vi "Get Joystick 2016.vi"() -> (2 "Pilot-CoPilot Controls":T1)   [LabVIEW 2015]
uses:
  Subsystem VIs/Robot Control Outputs 2016.ctl
  Global Variables/refnum names.vi
  <vilib>/Rock Robotics/WPI/Utilities/WPI_GetSetVariantRefNum.vi
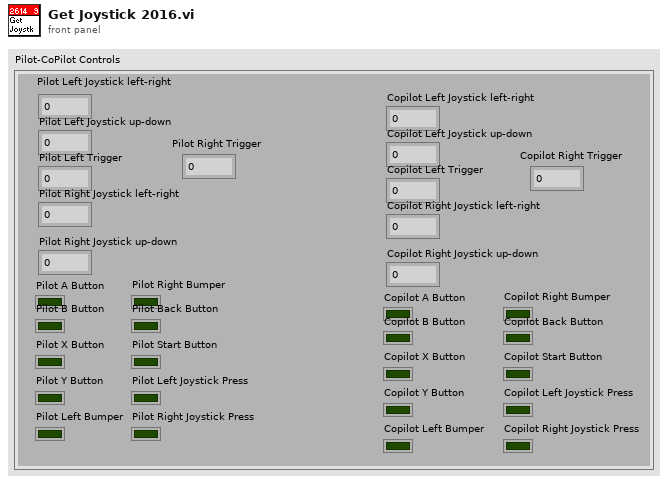
[diagram p1: front panel]
types:
  T1 = typedef "Robot Control Outputs 2016.ctl" = cluster{"Pilot Left Joystick left-right":dbl, "Pilot Left Joystick up-down":dbl, "Pilot A Button":bool, "Pilot B Button":bool, "Pilot X Button":bool, "Pilot Y Button":bool, "Pilot Left Bumper":bool, "Pilot Right Bumper":bool, "Pilot Back Button":bool, "Pilot Start Button":bool, "Pilot Left Joystick Press":bool, "Pilot Right Joystick Press":bool, "Pilot Left Trigger":dbl, "Pilot Right Joystick left-right":dbl, "Pilot Right Joystick up-down":dbl, "Pilot Right Trigger":dbl, "Copilot Left Joystick left-right":dbl, "Copilot Left Joystick up-down":dbl, "Copilot A Button":bool, "Copilot B Button":bool, "Copilot X Button":bool, "Copilot Y Button":bool, "Copilot Left Bumper":bool, "Copilot Right Bumper":bool, "Copilot Back Button":bool, "Copilot Start Button":bool, "Copilot Left Joystick Press":bool, "Copilot Right Joystick Press":bool, "Copilot Left Trigger":dbl, "Copilot Right Joystick left-right":dbl, "Copilot Right Joystick up-down":dbl, "Copilot Right Trigger":dbl}
  T2 = typedef "WPI_JoystickDevRef.ctl" = cluster{"Device":T3}
  T3 = typedef "WPI_JoystickDeviceEnum.ctl" = enum16{"USB 0", "USB 1", "USB 2", "USB 3", "USB 4", "USB 5"}
  T4 = cluster{"Axes[0]":dbl, "Axes[1]":dbl, "Axes[2]":dbl, "Axes[3]":dbl, "Axes[4]":dbl, "Axes[5]":dbl, "Axes[6]":dbl, "Axes[7]":dbl, "Axes[8]":dbl}
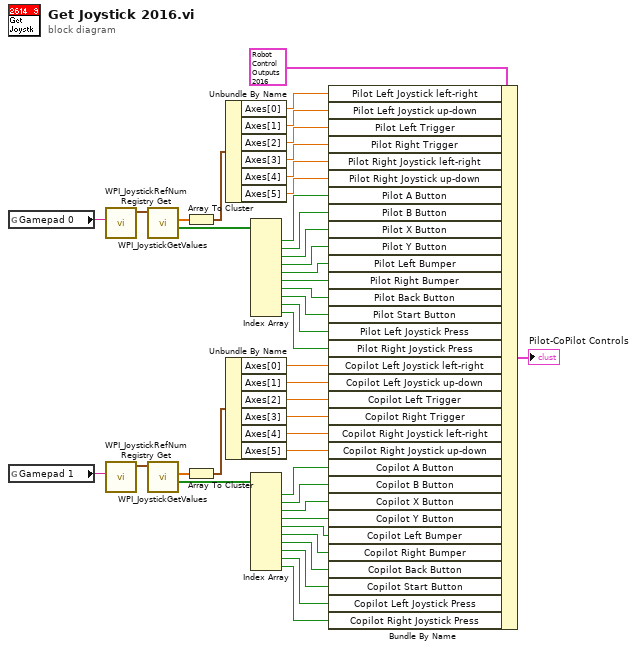
[diagram p0: block diagram]
diagram:
  n1 = global read "refnum names.vi" "Gamepad 0"() -> (w21:string)
  n2 = global read "refnum names.vi" "Gamepad 1"() -> (w20:string)
  n3 = call <vilib>:"WPI_JoystickRefNum Registry Get.vi"("refnum name"=w21) -> ("JoystickDevRef"=w42:T2)  [unwired: 9 in, 1 out]
  n4 = call <vilib>:"WPI_JoystickRefNum Registry Get.vi"("refnum name"=w20) -> ("JoystickDevRef"=w22:T2)  [unwired: 9 in, 1 out]
  n5 = call <vilib>:"WPI_JoystickGetValues.vi"("JoystickDevRef"=w42) -> ("Buttons"=w33:bool[], "Axes"=w41:dbl[])  [unwired: 6 in, 3 out]
  n6 = call <vilib>:"WPI_JoystickGetValues.vi"("JoystickDevRef"=w22) -> ("Buttons"=w18:bool[], "Axes"=w19:dbl[])  [unwired: 6 in, 3 out]
  n7 = Array To Cluster(array=w41) -> (cluster=w40:T4)
  n8 = Array To Cluster(array=w19) -> (cluster=w17:T4)
  n9 = Unbundle By Name(w40) -> ("Axes[0]"=w39:dbl, "Axes[1]"=w38:dbl, "Axes[2]"=w37:dbl, "Axes[3]"=w36:dbl, "Axes[4]"=w35:dbl, "Axes[5]"=w34:dbl)
  n10 = Unbundle By Name(w17) -> ("Axes[0]"=w16:dbl, "Axes[1]"=w15:dbl, "Axes[2]"=w14:dbl, "Axes[3]"=w13:dbl, "Axes[4]"=w12:dbl, "Axes[5]"=w11:dbl)
  n11 = Index Array(array=w33) -> (element #1=w32:bool, element #2=w31:bool, element #3=w30:bool, element #4=w29:bool, element #5=w28:bool, element #6=w27:bool, element #7=w26:bool, element #8=w25:bool, element #9=w24:bool, element #10=w23:bool)  [unwired: 10 in]
  n12 = Index Array(array=w18) -> (element #1=w10:bool, element #2=w9:bool, element #3=w8:bool, element #4=w7:bool, element #5=w5:bool, element #6=w6:bool, element #7=w4:bool, element #8=w3:bool, element #9=w2:bool, element #10=w1:bool)  [unwired: 10 in]
  n13 = Bundle By Name(cluster=T1 {"Pilot Left Joystick left-right"=0.0, "Pilot Left Joystick up-down"=0.0, "Pilot A Button"=FALSE, "Pilot B Button"=FALSE, "Pilot X Button"=FALSE, "Pilot Y Button"=FALSE, "Pilot Left Bumper"=FALSE, "Pilot Right Bumper"=FALSE, "Pilot Back Button"=FALSE, "Pilot Start Button"=FALSE, "Pilot Left Joystick Press"=FALSE, "Pilot Right Joystick Press"=FALSE, "Pilot Left Trigger"=0.0, "Pilot Right Joystick left-right"=0.0, "Pilot Right Joystick up-down"=0.0, "Pilot Right Trigger"=0.0, "Copilot Left Joystick left-right"=0.0, "Copilot Left Joystick up-down"=0.0, "Copilot A Button"=FALSE, "Copilot B Button"=FALSE, "Copilot X Button"=FALSE, "Copilot Y Button"=FALSE, "Copilot Left Bumper"=FALSE, "Copilot Right Bumper"=FALSE, "Copilot Back Button"=FALSE, "Copilot Start Button"=FALSE, "Copilot Left Joystick Press"=FALSE, "Copilot Right Joystick Press"=FALSE, "Copilot Left Trigger"=0.0, "Copilot Right Joystick left-right"=0.0, "Copilot Right Joystick up-down"=0.0, "Copilot Right Trigger"=0.0} ("Pilot-CoPilot Controls"), "Pilot Left Joystick left-right"=w39, "Pilot Left Joystick up-down"=w38, "Pilot Left Trigger"=w37, "Pilot Right Trigger"=w36, "Pilot Right Joystick left-right"=w35, "Pilot Right Joystick up-down"=w34, "Pilot A Button"=w32, "Pilot B Button"=w31, "Pilot X Button"=w30, "Pilot Y Button"=w29, "Pilot Left Bumper"=w28, "Pilot Right Bumper"=w27, "Pilot Back Button"=w26, "Pilot Start Button"=w25, "Pilot Left Joystick Press"=w24, "Pilot Right Joystick Press"=w23, "Copilot Left Joystick left-right"=w16, "Copilot Left Joystick up-down"=w15, "Copilot Left Trigger"=w14, "Copilot Right Trigger"=w13, "Copilot Right Joystick left-right"=w12, "Copilot Right Joystick up-down"=w11, "Copilot A Button"=w10, "Copilot B Button"=w9, "Copilot X Button"=w8, "Copilot Y Button"=w7, "Copilot Left Bumper"=w5, "Copilot Right Bumper"=w6, "Copilot Back Button"=w4, "Copilot Start Button"=w3, "Copilot Left Joystick Press"=w2, "Copilot Right Joystick Press"=w1) -> (→"Pilot-CoPilot Controls":T1)
